vi "Configure PLL Mode.vi"(8 "error in (no error)":errorcluster, 10 "PLL Mode":T1, 11 "SA-ESA in":refnum<class "SA-ESA.lvclass">) -> (0 "error out":errorcluster, 3 "SA-ESA out":refnum<class "SA-ESA.lvclass">)   [LabVIEW 2020, in "SA-ESA.lvclass"]
uses:
  SA-ESA.lvclass
  Controls/PLL Mode.ctl
  Spectrum Analyzer.lvclass
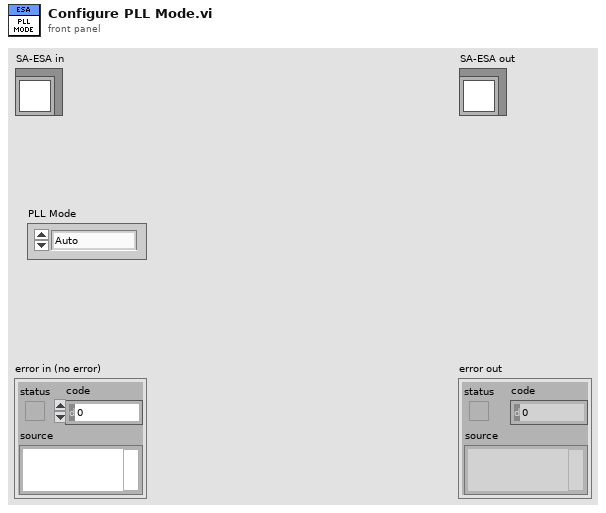
[diagram p1: front panel]
types:
  T1 = typedef "Spectrum Analyzer.lvclass/PLL Mode.ctl" = enum16{"Auto", "Narrow", "Normal", "Wide"}
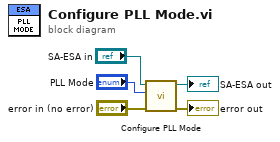
[diagram p0: block diagram]
diagram:
  n1 = call-parent "Configure PLL Mode.vi"("error in (no error)"="error in (no error)", "PLL Mode"="PLL Mode", "Spectrum Analyzer in"="SA-ESA in") -> ("error out"=→"error out":errorcluster, "Spectrum Analyzer out"=→"SA-ESA out":refnum<class "SA-ESA.lvclass">)  [unwired: 7 in]
